vi "SaveAsXLS.vi"(9 "Data Table":string[][](table), 11 "file":path) -> ()   [LabVIEW 2022 SP3]
uses:
  <vilib>/express/express shared/NI_ExcelFile/Ctrls/FileOperation.ctl
  <vilib>/express/express shared/NI_ExcelFile/SubVIs/WriteData (Array of STR).vi
  <vilib>/express/express shared/NI_ExcelFile/NI_ExcelFile.lvlib
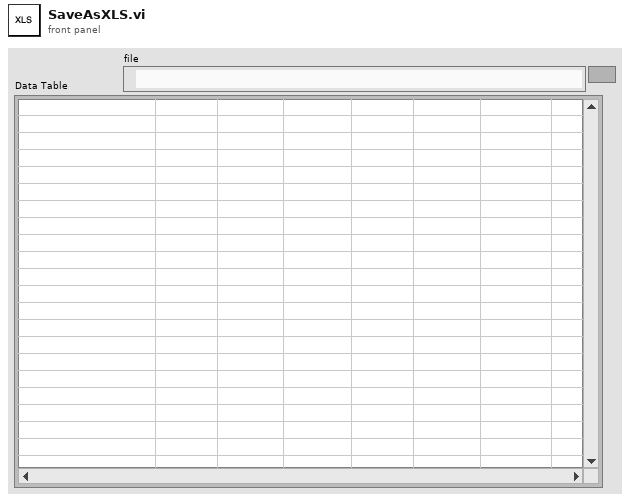
[diagram p1: front panel]
types:
  T1 = typedef "NI_ExcelFile.lvlib/FileOperation.ctl" = enum16{"open or create", "open", "create or replace", "create"}
  T2 = typedef "NI_ExcelFile.lvlib/ExcelRefnum.ctl" = refnum<data-value>
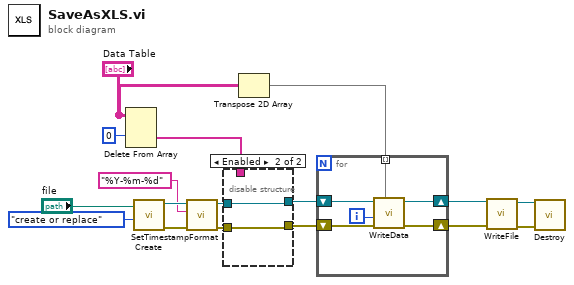
[diagram p0: block diagram]
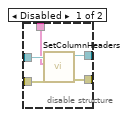
[diagram p2: hidden frame]
diagram:
  n1 = Delete From Array(array="Data Table", index (row)=0) -> (deleted portion=w11:string[])  [unwired: 2 in, 1 out]
  n2 = call <vilib>:"Create.vi"("operation (0: open or create)"=FileOperation."create or replace", "file"="file") -> ("error out"=w15:errorcluster, "Excel refnum out"=w17:T2)  [unwired: 8 in]
  n3 = call <vilib>:"SetTimestampFormat.vi"("error in (no error)"=w15, "timestamp format"="%Y-%m-%d", "Excel refnum"=w17) -> ("error out"=w4:errorcluster, "Excel refnum out"=w14:T2)  [unwired: 7 in]
  n4 = disable-structure shown="Enabled" {
    disable-tunnel: w14 -> [w22 w24]
    disable-tunnel: [w21 w24] -> w13
    disable-tunnel: w11 -> [w20 _]
    disable-tunnel: [w19 w23] -> w10
    disable-tunnel: w4 -> [w18 w23]
    frame Disabled {
      n5 = call <vilib>:"SetColumnHeaders.vi"("error in (no error)"=w18, "column headers"=w20, "Excel refnum"=w22) -> ("error out"=w19:errorcluster, "Excel refnum out"=w21:T2)  [unwired: 7 in]
    }
    frame Enabled {
    }
  }
  n6 = Transpose 2D Array(2D array="Data Table") -> (transposed array=w2:string[][])
  n7 = for {
    tunnel: w2 -> [w26] mode=indexing
    shift-right: [w28] -> w9
    shift-left: w13 -> [w30]
    shift-right: [w27] -> w8
    shift-left: w10 -> [w29]
    i -> [w25]
    n8 = call-poly <vilib>:"WriteData.vi"("Array of STR"=w26, "error in (no error)"=w29, "channel index (0)"=w25, "Excel refnum"=w30) -> ("error out"=w27:errorcluster, "Excel refnum out"=w28:T2)  [unwired: 6 in]
  }
  n9 = call <vilib>:"WriteFile.vi"("error in (no error)"=w8, "Excel refnum"=w9) -> ("error out"=w6:errorcluster, "Excel refnum out"=w7:T2)  [unwired: 8 in]
  n10 = call <vilib>:"Destroy.vi"("error in (no error)"=w6, "Excel refnum"=w7) -> ()  [unwired: 8 in, 2 out]
